vi "Register Dynamic Events.vi"(8 "error in (no error)":errorcluster, 11 "ControlEventHandler In":refnum<class "ControlEventHandler.lvclass">) -> (0 "error out":errorcluster, 3 "ControlEventHandler Out":refnum<class "ControlEventHandler.lvclass">)   [LabVIEW 2020, in "ActorEvents.lvlib" / "ControlEventHandler.lvclass"]
uses:
  <vilib>/gpm_packages/@cs/mva-viewable/Source/ActorEvents/EventHandler/ControlEventHandler/ControlEventHandler.lvclass
  C:/Program Files/National Instruments/LabVIEW 2020/vi.lib/gpm_packages/@cs/mva-viewable/Source/ActorEvents/IEventHandler/IEventHandler.lvclass
  <vilib>/gpm_packages/@cs/mva-viewable/Source/ActorEvents/IEventHandler/IEventHandler.lvclass/IEventHandler.ctl
  <vilib>/event_ctls.llb/lveventtype.ctl
  <vilib>/gpm_packages/@cs/mva-viewable/Source/ActorEvents/EventHandler/ControlEventHandler/ControlEventHandler.lvclass/ControlEventHandler.ctl
  <vilib>/gpm_packages/@cs/mva-viewable/Source/ActorEvents/IEventHandler/Read Registrations.vi
  <vilib>/gpm_packages/@cs/mva-viewable/Source/ActorEvents/IEventHandler/IEventHandler.lvclass
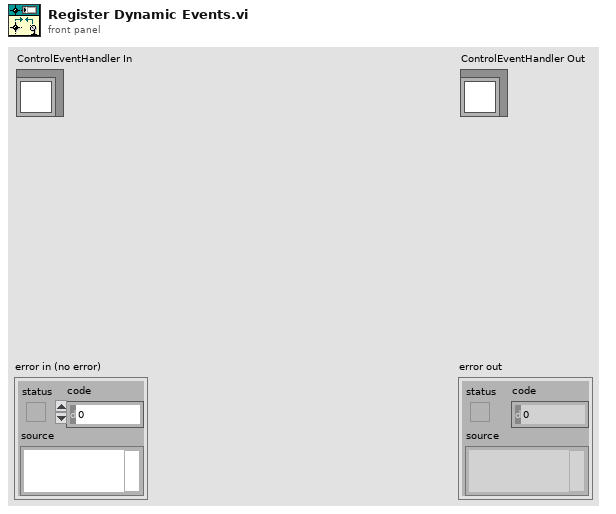
[diagram p1: front panel]
types:
  T1 = typedef "lveventtype.ctl" = enum32{"Null", "Timeout", "Annotation Menu Selection", "Annotation Menu Selection?", "App Instance Close", "App Instance Close?", "Autoscale Range Change", "Bookmark Info Change", "Cell Edit", "Cell Edit?", "Cursor Grab", "Cursor Grab?", "Cursor Menu Selection", "Cursor Menu Selection?", "Cursor Move", "Cursor Release", "Data Change", "Direction Change", "Display State Change", "Drag Ended", "Drag Enter", "Drag Leave", "Drag Over", "Drag Source Update", "Drag Starting", "Drag Starting?", "Drop", "Exec State Change", "Key Down", "Key Down?", "Key Repeat", "Key Repeat?", "Key Up", "Listbox Double Click", "Menu Activation?", "Menu Selection (App)", "Menu Selection? (App)", "Menu Selection (User)", "Mouse Down", "Mouse Down?", "Mouse Enter", "Mouse Leave", "Mouse Move", "Mouse Up", "Mouse Wheel", "NI Security User Change (App)", "Pane Size", "Panel Close", "Panel Close?", "Panel Resize", "Plot Attribute Change", "Scale Range Change", "Shortcut Menu Activation?", "Shortcut Menu Selection (App)", "Shortcut Menu Selection? (App)", "Shortcut Menu Selection (User)", "Tree Double Click", "Tree Drag", "Tree Drag?", "Tree Drop", "Tree Drop?", "Tree Item Close", "Tree Item Close?", "Tree Item Open", "Tree Item Open?", "User Event", "Value Change"}
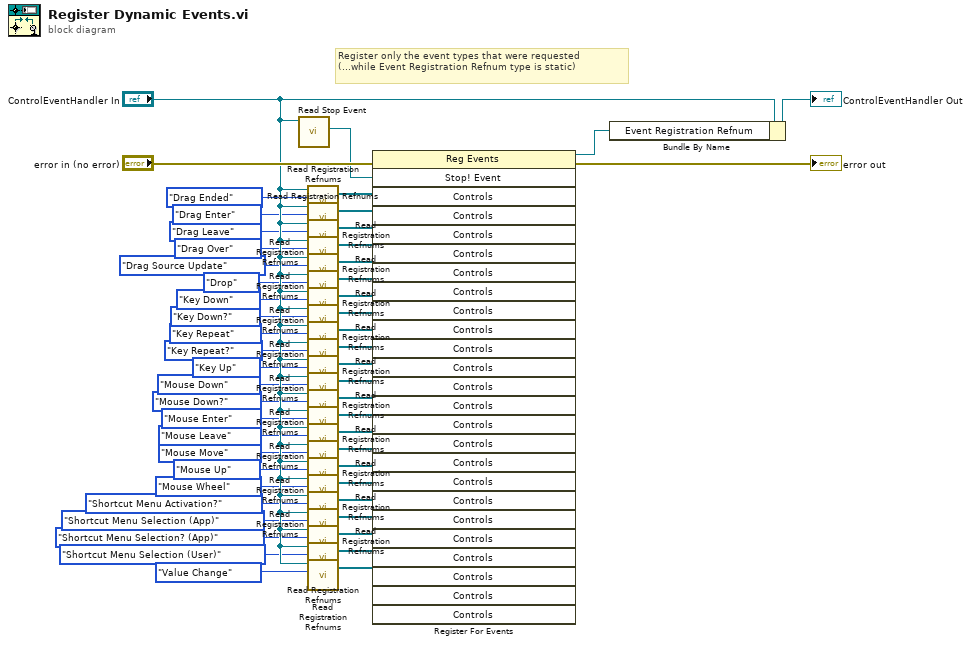
[diagram p0: block diagram]
diagram:
  # "Register only the event types that were requested\n(...while Event Registration Refnum type is static)"
  n1 = call <vilib>:"Read Stop Event.vi"("IEventHandler in"="ControlEventHandler In") -> ("Stop! Event"=w49:refnum<user-event>)  [unwired: 10 in]
  n2 = call <vilib>:"Read Registration Refnums.vi"("Event Type"=lveventtype."Drag Ended", "ControlEventHandler"="ControlEventHandler In") -> ("Controls"=w45:refnum<vi>[])  [unwired: 5 in]
  n3 = call <vilib>:"Read Registration Refnums.vi"("Event Type"=lveventtype."Drag Enter", "ControlEventHandler"="ControlEventHandler In") -> ("Controls"=w44:refnum<vi>[])  [unwired: 5 in]
  n4 = call <vilib>:"Read Registration Refnums.vi"("Event Type"=lveventtype."Drag Leave", "ControlEventHandler"="ControlEventHandler In") -> ("Controls"=w43:refnum<vi>[])  [unwired: 5 in]
  n5 = call <vilib>:"Read Registration Refnums.vi"("Event Type"=lveventtype."Drag Over", "ControlEventHandler"="ControlEventHandler In") -> ("Controls"=w42:refnum<vi>[])  [unwired: 5 in]
  n6 = call <vilib>:"Read Registration Refnums.vi"("Event Type"=lveventtype."Drag Source Update", "ControlEventHandler"="ControlEventHandler In") -> ("Controls"=w41:refnum<vi>[])  [unwired: 5 in]
  n7 = call <vilib>:"Read Registration Refnums.vi"("Event Type"=lveventtype."Drop", "ControlEventHandler"="ControlEventHandler In") -> ("Controls"=w40:refnum<vi>[])  [unwired: 5 in]
  n8 = call <vilib>:"Read Registration Refnums.vi"("Event Type"=lveventtype."Key Down", "ControlEventHandler"="ControlEventHandler In") -> ("Controls"=w39:refnum<vi>[])  [unwired: 5 in]
  n9 = call <vilib>:"Read Registration Refnums.vi"("Event Type"=lveventtype."Key Down?", "ControlEventHandler"="ControlEventHandler In") -> ("Controls"=w38:refnum<vi>[])  [unwired: 5 in]
  n10 = call <vilib>:"Read Registration Refnums.vi"("Event Type"=lveventtype."Key Repeat", "ControlEventHandler"="ControlEventHandler In") -> ("Controls"=w37:refnum<vi>[])  [unwired: 5 in]
  n11 = call <vilib>:"Read Registration Refnums.vi"("Event Type"=lveventtype."Key Repeat?", "ControlEventHandler"="ControlEventHandler In") -> ("Controls"=w36:refnum<vi>[])  [unwired: 5 in]
  n12 = call <vilib>:"Read Registration Refnums.vi"("Event Type"=lveventtype."Key Up", "ControlEventHandler"="ControlEventHandler In") -> ("Controls"=w35:refnum<vi>[])  [unwired: 5 in]
  n13 = call <vilib>:"Read Registration Refnums.vi"("Event Type"=lveventtype."Mouse Down", "ControlEventHandler"="ControlEventHandler In") -> ("Controls"=w34:refnum<vi>[])  [unwired: 5 in]
  n14 = call <vilib>:"Read Registration Refnums.vi"("Event Type"=lveventtype."Mouse Down?", "ControlEventHandler"="ControlEventHandler In") -> ("Controls"=w33:refnum<vi>[])  [unwired: 5 in]
  n15 = call <vilib>:"Read Registration Refnums.vi"("Event Type"=lveventtype."Mouse Enter", "ControlEventHandler"="ControlEventHandler In") -> ("Controls"=w32:refnum<vi>[])  [unwired: 5 in]
  n16 = call <vilib>:"Read Registration Refnums.vi"("Event Type"=lveventtype."Mouse Leave", "ControlEventHandler"="ControlEventHandler In") -> ("Controls"=w31:refnum<vi>[])  [unwired: 5 in]
  n17 = call <vilib>:"Read Registration Refnums.vi"("Event Type"=lveventtype."Mouse Move", "ControlEventHandler"="ControlEventHandler In") -> ("Controls"=w30:refnum<vi>[])  [unwired: 5 in]
  n18 = call <vilib>:"Read Registration Refnums.vi"("Event Type"=lveventtype."Mouse Up", "ControlEventHandler"="ControlEventHandler In") -> ("Controls"=w29:refnum<vi>[])  [unwired: 5 in]
  n19 = call <vilib>:"Read Registration Refnums.vi"("Event Type"=lveventtype."Mouse Wheel", "ControlEventHandler"="ControlEventHandler In") -> ("Controls"=w28:refnum<vi>[])  [unwired: 5 in]
  n20 = call <vilib>:"Read Registration Refnums.vi"("Event Type"=lveventtype."Shortcut Menu Activation?", "ControlEventHandler"="ControlEventHandler In") -> ("Controls"=w27:refnum<vi>[])  [unwired: 5 in]
  n21 = call <vilib>:"Read Registration Refnums.vi"("Event Type"=lveventtype."Shortcut Menu Selection (App)", "ControlEventHandler"="ControlEventHandler In") -> ("Controls"=w26:refnum<vi>[])  [unwired: 5 in]
  n22 = call <vilib>:"Read Registration Refnums.vi"("Event Type"=lveventtype."Shortcut Menu Selection? (App)", "ControlEventHandler"="ControlEventHandler In") -> ("Controls"=w25:refnum<vi>[])  [unwired: 5 in]
  n23 = call <vilib>:"Read Registration Refnums.vi"("Event Type"=lveventtype."Shortcut Menu Selection (User)", "ControlEventHandler"="ControlEventHandler In") -> ("Controls"=w24:refnum<vi>[])  [unwired: 5 in]
  n24 = call <vilib>:"Read Registration Refnums.vi"("Event Type"=lveventtype."Value Change", "ControlEventHandler"="ControlEventHandler In") -> ("Controls"=w47:refnum<vi>[])  [unwired: 5 in]
  n25 = register-events(error in="error in (no error)", w49, w45, w44, w43, w42, w41, w40, w39, w38, w37, w36, w35, w34, w33, w32, w31, w30, w29, w28, w27, w26, w25, w24, w47) -> (reference out=w46:refnum<event-registration>, error out=→"error out":errorcluster)  [unwired: 1 in]
  n26 = Bundle By Name(cluster="ControlEventHandler In", "Event Registration Refnum"=w46) -> (→"ControlEventHandler Out":refnum<class "ControlEventHandler.lvclass">)
